vi "memo_ta_array_admin.vi"(11 "Cluster":T1) -> (3 "appended array":u32[](array[numeric]))   [LabVIEW 2015, in "PolyVIEW.lvclass"]
uses:
  PolyVIEW.lvclass
  Admin memo.ctl
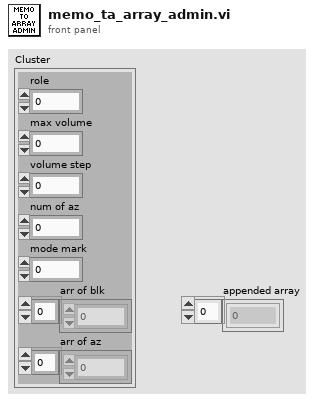
[diagram p1: front panel]
types:
  T1 = typedef "Admin memo.ctl" = cluster{"role":i32, "max volume":i32, "volume step":i32, "num of az":i32, "mode mark":i32, "arr of blk":i32[], "arr of az":i32[]}
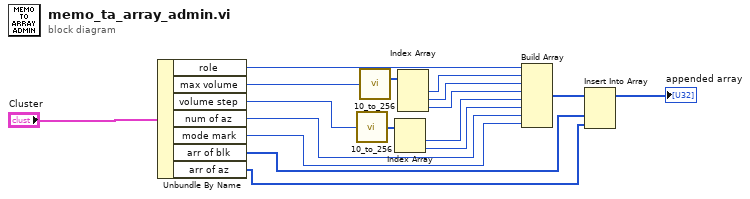
[diagram p0: block diagram]
diagram:
  n1 = Unbundle By Name("Cluster") -> ("role"=w17:i32, "max volume"=w13:i32, "volume step"=w9:i32, "num of az"=w6:i32, "mode mark"=w5:i32, "arr of blk"=w2:i32[], "arr of az"=w1:i32[])
  n2 = call "10_to_256.vi"("Decimal"=w9) -> ("256"=w15:u8[])
  n3 = call "10_to_256.vi"("Decimal"=w13) -> ("256"=w16:u8[])
  n4 = Index Array(array=w15) -> (element #1=w8:u8, element #2=w7:u8)  [unwired: 2 in]
  n5 = Index Array(array=w16) -> (element #1=w12:u8, element #2=w11:u8, element #3=w10:u8)  [unwired: 3 in]
  n6 = Build Array(w17, w12, w11, w10, w8, w7, w6, w5) -> (w4:i32[])
  n7 = Insert Into Array(array=w4, new element #1=w2, new element #2=w1) -> (→"appended array":i32[])  [unwired: 1 in]
